vi "setUp.vi"(8 "error in (no error)":errorcluster, 11 "reference in":refnum<class "TestCase.Pointer.lvclass">) -> (0 "error out":errorcluster, 3 "reference out":refnum<class "TestCase.Pointer.lvclass">)   [LabVIEW 2016, in "TestCase.Pointer.lvclass"]
doc: "setUp runs prior to the test method during test execution. Use this method to initialize any object data required by your tests."
uses:
  TestCase.Pointer.lvclass
  C:/Program Files (x86)/National Instruments/LabVIEW 2016/vi.lib/addons/_JKI Toolkits/VI Tester/TestCase.llb/TestCase.lvclass
  Source/Classes/Pointer/Pointer.lvclass
  TestCase.Pointer.lvclass/TestCase.Pointer.ctl
  Source/Classes/Pointer/New (1B).vi
  <vilib>/addons/_JKI Toolkits/VI Tester/TestCase.llb/TestCase.lvclass
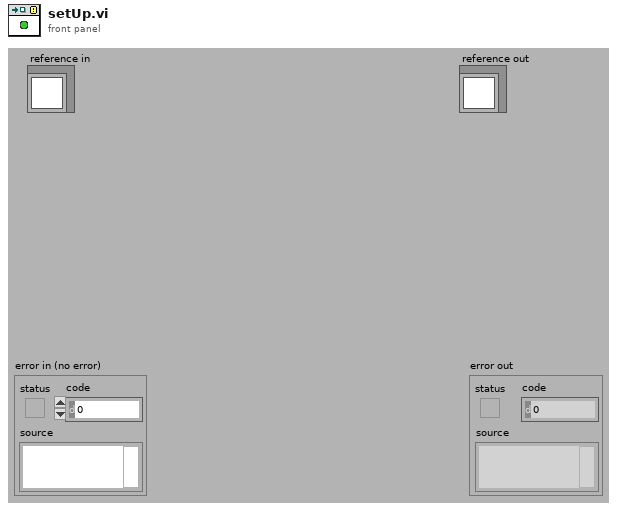
[diagram p1: front panel]
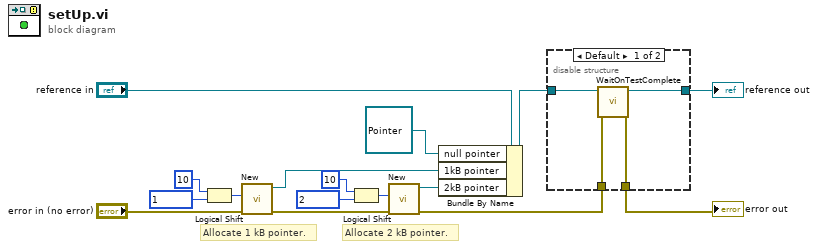
[diagram p0: block diagram]
diagram:
  # "Allocate 1 kB pointer."
  # "Allocate 2 kB pointer."
  n1 = Logical Shift(y=i16 10, x=u64 1 ("size")) -> (x << y=w7:u64)
  n2 = call-poly "New.vi"("error in (no error)"="error in (no error)", "count (1)"=w7) -> ("error out"=w5:errorcluster, "Pointer"=w4:refnum<class "Pointer.lvclass">)  [unwired: 8 in]
  n3 = Logical Shift(y=i16 10, x=u64 2 ("size")) -> (x << y=w11:u64)
  n4 = call-poly "New.vi"("error in (no error)"=w5, "count (1)"=w11) -> ("error out"=w2:errorcluster, "Pointer"=w10:refnum<class "Pointer.lvclass">)  [unwired: 8 in]
  n5 = Bundle By Name(cluster="reference in", "null pointer"=refnum<class "Pointer.lvclass"> refnum, "1kB pointer"=w4, "2kB pointer"=w10) -> (w14:refnum<class "TestCase.Pointer.lvclass">)
  n6 = disable-structure shown="Default" {
    disable-tunnel: w2 -> [w20 w21]
    disable-tunnel: [w19 w21] -> w16
    disable-tunnel: [w18 w22] -> w15
    disable-tunnel: w14 -> [w17 w22]
    frame condition #0 (active) {
      n7 = call <vilib>:"WaitOnTestComplete.vi"("error in (no error)"=w20, "TestCase in"=w17) -> ("error out"=w19:errorcluster, "TestCase out"=w18:refnum<class "TestCase.Pointer.lvclass">)  [unwired: 8 in]
    }
    frame condition #1 {
    }
  }
  "error out" <- w16
  "reference out" <- w15
